vi "get_parameter_debug.vi"(6 "timeout (25000ms)":i32=25000, 8 "error in (no error)":errorcluster, 10 "array":string[](array[string]), 11 "daemon reference in":refnum<k5>) -> (0 "error out":errorcluster, 2 "values":u8[](array[numeric]), 3 "daemon reference out":refnum<k5>, 5 "command out":string="random")   [LabVIEW 2017]
doc: "<b>Command: </b>\"get_parameter\"\n\n<b>Description: </b> Instructs the target to return the specified parameter values.\n\n<b>Parameters: </b> \n\n 1. Parameter Array [max 20]\n____________________________________________\nDIPC 692 Daemon API 10.0.0.1\nSam Tee - Dyson Technology Ltd\nCopyright (c) 2024, Dyson Technology Ltd"
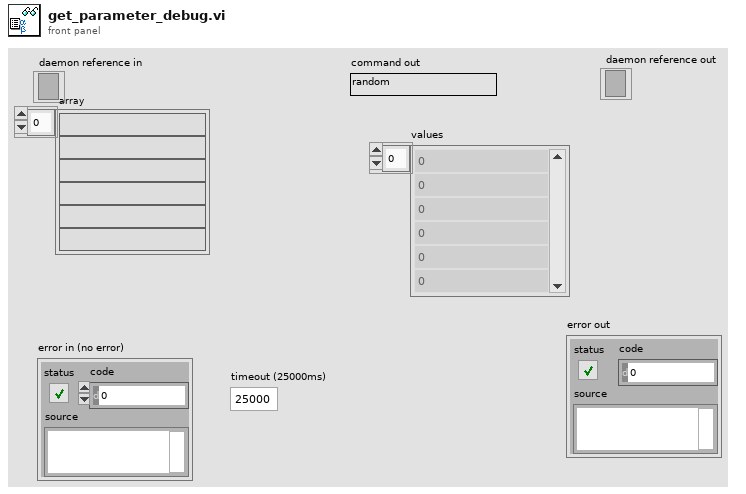
[diagram p1: front panel]
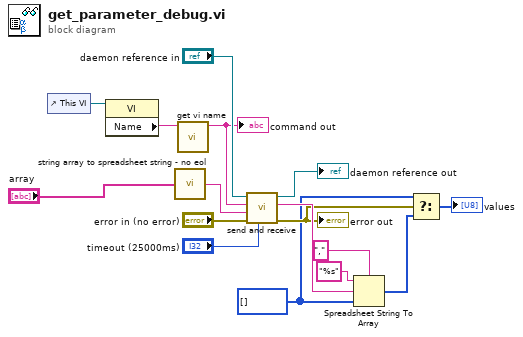
[diagram p0: block diagram]
diagram:
  w4 = u8[] []
  n1 = control-ref of="This VI"() -> (w12:refnum<vi>)
  n2 = property class="VI"(reference=w12) -> ("Name"=w11:string)  [unwired: 1 in, 2 out]
  n3 = call "string array to spreadsheet string - no eol.vi"("string array"="array") -> ("spreadsheet string - no eol"=w6:string)
  n4 = call "get vi name.vi"("library.lvlib:name.vi"=w11) -> ("vi name"=w10:string)  [unwired: 10 in]
  "command out" <- w10
  n5 = call "send and receive.vi"("timeout (25000ms)"="timeout (25000ms)", "error in (no error)"="error in (no error)", "data"=w6, "command"=w10, "daemon reference in"="daemon reference in") -> ("error out"=w5:errorcluster, "response"=w9:string, "daemon reference out"=→"daemon reference out":refnum<k5>)  [unwired: 4 in]
  "error out" <- w5
  n6 = Spreadsheet String To Array(delimiter (Tab)=",", format string="%s", spreadsheet string=w9, array type (2D Dbl)=w4) -> (array=w3:u8[])
  n7 = Select(t=w4, s=w5, f=w3) -> (s? t:f=→"values":u8[])
